vi "thresh_diff.vi"(10 "diff_thresh":fxp<+/-,16,8>, 11 "x_diff in":fxp<+/-,16,8>) -> (3 "thresh_out":fxp<+/-,16,8>)   [LabVIEW 2020]
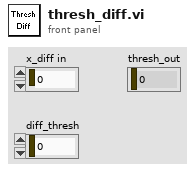
[diagram p1: front panel]
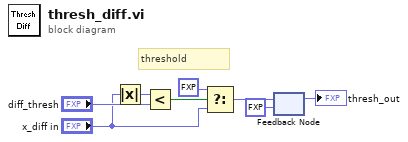
[diagram p0: block diagram]
diagram:
  # "threshold"
  n1 = Absolute Value(x="x_diff in") -> (abs(x)=w2:fxp<+,16,8>)
  n2 = Less?(x=w2, y="diff_thresh") -> (x < y?=w3:bool)
  n3 = Select(t=fxp<+/-,16,8> data[17B], s=w3, f="x_diff in") -> (s? t:f=w4:fxp<+/-,16,8>)
  n4 = feedback #1(fxp<+/-,16,8> data[17B] ("x_diff 2")) -> (→"thresh_out":fxp<+/-,16,8>)
  n5 = feedback-in #1(w4) -> ()
